vi "kvCanGetBusOutputControl.vi"(0 "Channel Handle (input only)":i32, 1 "error in (no error)":errorcluster) -> (2 "Channel Handle (ouput only)":i32, 3 "Normal Driver Mode":bool, 4 "Silent Driver Mode":bool, 5 "error out":errorcluster)   [LabVIEW 2022 SP3]
doc: "This function retrieves the current CAN controller driver type. This corresponds loosely to the bus output control register in the CAN controller, hence the name of this function. CANLIB32 does not allow for direct manipulation of the bus output control register; instead, symbolic constants are used to select the desired driver type."
uses:
  canlib32.dll
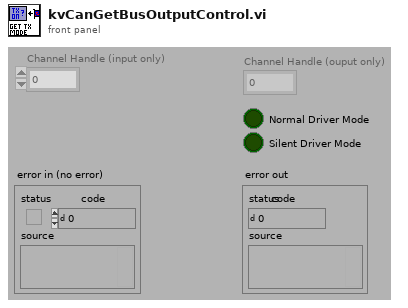
[diagram p1: front panel]
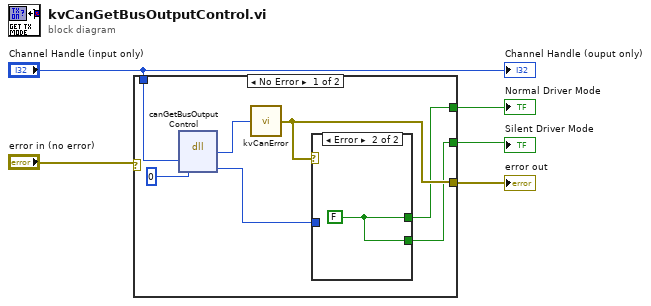
[diagram p0: block diagram]
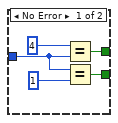
[diagram p2: hidden frame]
diagram:
  n1 = case shown="No Error" "error in (no error)" {
    selector: "error in (no error)" -> [_ w20]
    tunnel: [w9 w20] -> w4
    tunnel: "Channel Handle (input only)" -> [w12 _]
    tunnel: [w8 w19] -> w2
    tunnel: [w7 w19] -> w1
    frame No Error {
      n2 = dll-call lib="canlib32.dll" fn="canGetBusOutputControl"("hnd"=w12, "drivertype"=0) -> (w10:i32, "drivertype"=w6:u32)  [unwired: 4 in, 2 out]
      n3 = call "kvCanError.vi"("error code"=w10) -> ("error out"=w9:errorcluster)
      n4 = case shown="Error" w9 {
        tunnel: [w16 w18] -> w8
        tunnel: [w17 w18] -> w7
        tunnel: w6 -> [w15 _]
        frame No Error {
          n5 = Equal?(x=4, y=w15) -> (x = y?=w16:bool)
          n6 = Equal?(x=w15, y=1) -> (x = y?=w17:bool)
        }
        frame Error {
          w18 = FALSE
        }
      }
    }
    frame Error {
      w19 = FALSE
    }
  }
  "error out" <- w4
  "Normal Driver Mode" <- w2
  "Silent Driver Mode" <- w1
  "Channel Handle (ouput only)" <- "Channel Handle (input only)"
